vi "Panel.vi"(11 "ExBlank in":refnum<class "ExBlank.lvclass">) -> ()   [LabVIEW 2020, in "2D Array Example.lvlib" / "ExBlank.lvclass"]
uses:
  ExBlank.lvclass
  C:/dev/lv20CE/lv-oopanel/OOPanel/Panel/Panel.lvclass
  OOPanel/Panel/Basic UI State.ctl
  OOPanel/Panel/Panel.lvclass
  OOPanel/OOPanel.lvlib
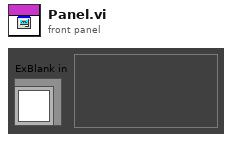
[diagram p1: front panel]
types:
  T1 = typedef "OOPanel.lvlib/Panel.lvclass/Basic UI State.ctl" = enum16{"Init", "Run", "Close"}
  T2 = typedef "OOPanel.lvlib/Panel.lvclass/Panel Events.ctl" = cluster{"Visbility":refnum<user-event>, "Close":refnum<user-event>}
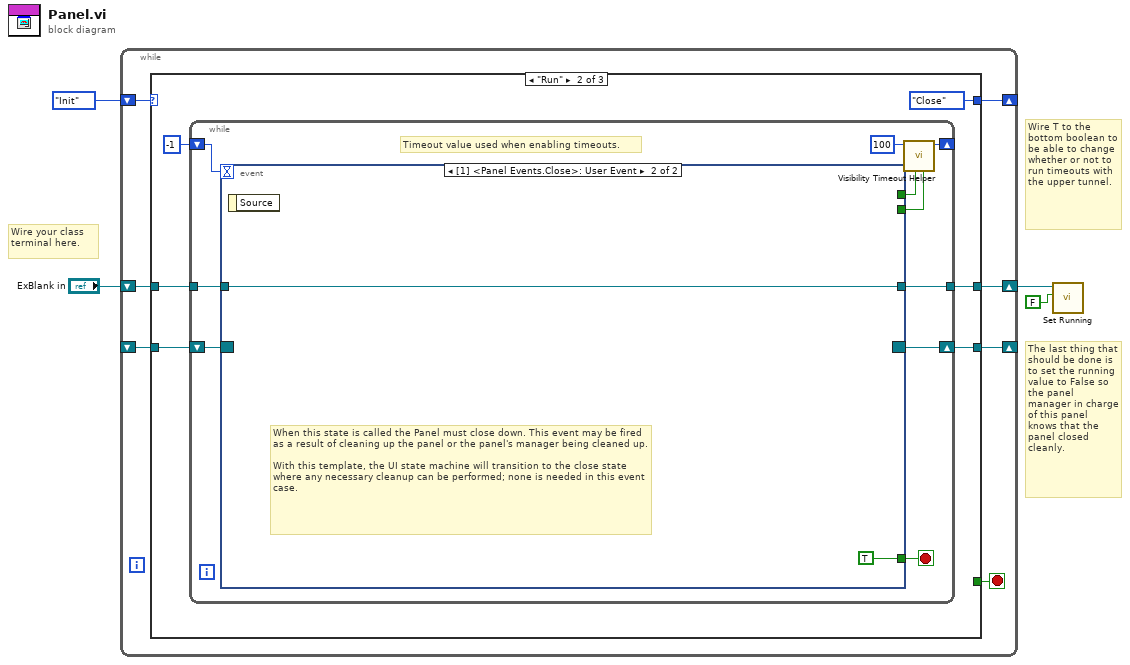
[diagram p0: block diagram]
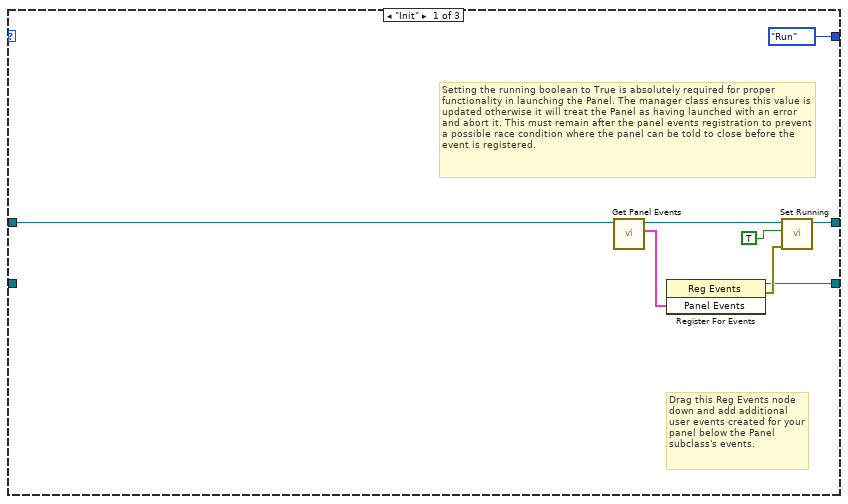
[diagram p2: hidden frame]
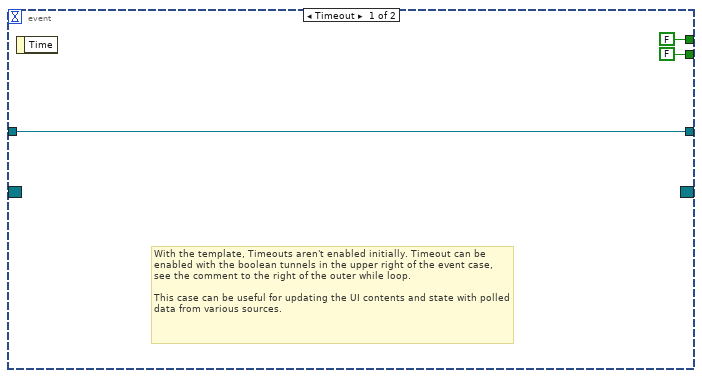
[diagram p3: hidden frame]
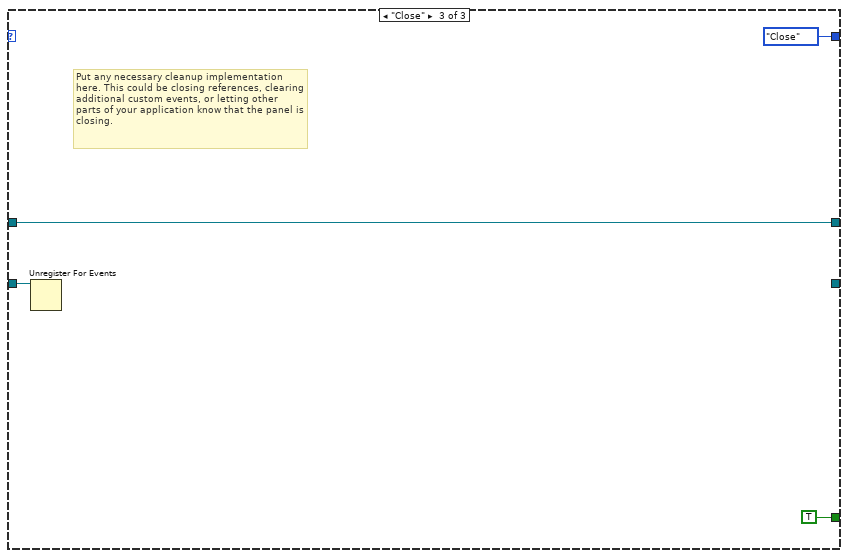
[diagram p4: hidden frame]
diagram:
  # "The last thing that should be done is to set the running value to False so the panel manager in charge of this panel knows that the panel closed cleanly."
  # "Wire T to the bottom boolean to be able to change whether or not to run timeouts with the upper tunnel."
  # "Wire your class terminal here."
  n1 = while {
    shift-right: [w10] -> _
    shift-left: _ -> [w11]
    shift-right: [w8] -> _
    shift-left: Basic_UI_State."Init" ("Basic UI State") -> [w9]
    shift-right: [w6] -> w4
    shift-left: "ExBlank in" -> [w5]
    stop <- w7 stop-if-true
    n2 = case shown="\"Run\"" w9 {
      tunnel: w11 -> [_ w25 w42]
      tunnel: [w16 w23 _] -> w10
      tunnel: [Basic_UI_State."Run" ("Basic UI State") Basic_UI_State."Close" ("Basic UI State") Basic_UI_State."Close" ("Basic UI State")] -> w8
      tunnel: [_ _ TRUE] -> w7
      tunnel: [w15 w20 w41] -> w6
      tunnel: w5 -> [w14 w21 w41]
      frame "Init" {
        # "Setting the running boolean to True is absolutely required for proper functionality in launching the Panel. The manager class ensures this value is updated otherwise it will treat the Panel as having launched with an error and abort it. This must remain after the panel events registration to prevent a possible race condition where the panel can be told to close before the event is registered."
        # "Drag this Reg Events node down and add additional user events created for your panel below the Panel subclass's events."
        n3 = call "Get Panel Events.vi"("Panel in"=w14) -> ("Panel Events"=w12:T2, "Panel out"=w13:refnum<class "ExBlank.lvclass">)  [unwired: 8 in, 1 out]
        n4 = register-events(w12) -> (reference out=w16:refnum<event-registration>, error out=w18:errorcluster)  [unwired: 2 in]
        n5 = call "Set Running.vi"("error in (no error)"=w18, "Running"=TRUE, "Panel in"=w13) -> ("Panel out"=w15:refnum<class "ExBlank.lvclass">)  [unwired: 7 in, 1 out]
      }
      frame "Run" {
        n6 = while {
          shift-right: [w31] -> w23
          shift-left: w25 -> [w32]
          shift-right: [w34] -> _
          shift-left: -1 ("Timeout") -> [w33]
          tunnel: w21 -> [w27]
          tunnel: [w26] -> w20
          stop <- w28 stop-if-true
          # "Timeout value used when enabling timeouts."
          n7 = event shown="[1] <Panel Events.Close>: User Event" {
            selector: w32 -> [_ _]
            dyn-events: [_ _] -> w31
            timeout: w33 -> [_ _]
            tunnel: [FALSE _] -> w30
            tunnel: [FALSE _] -> w29
            tunnel: [_ TRUE] -> w28
            tunnel: w27 -> [w36 w39]
            tunnel: [w36 w39] -> w26
            event Timeout {
              # "With the template, Timeouts aren't enabled initially. Timeout can be enabled with the boolean tunnels in the upper right of the event case, see the comment to the right of the outer while loop.\n\nThis case can be useful for updating the UI contents and state with polled data from various sources."
              n8 = event-data() -> ()  [unwired: 1 in, 1 out]
            }
            event User Event {
              # "When this state is called the Panel must close down. This event may be fired as a result of cleaning up the panel or the panel's manager being cleaned up.\n\nWith this template, the UI state machine will transition to the close state where any necessary cleanup can be performed; none is needed in this event case."
              n9 = event-data() -> ()  [unwired: 1 in, 1 out]
            }
          }
          n10 = call "Visibility Timeout Helper.vi"("Update?"=w29, "Use Timeout?"=w30, "Visible Timeout mS"=100) -> ("Timeout"=w34:i32)  [unwired: 8 in]
        }
      }
      frame "Close" {
        # "Put any necessary cleanup implementation here. This could be closing references, clearing additional custom events, or letting other parts of your application know that the panel is closing."
        n11 = Unregister For Events(event registration refnum=w42) -> ()  [unwired: 1 in, 1 out]
      }
    }
  }
  n12 = call "Set Running.vi"("Running"=FALSE, "Panel in"=w4) -> ()  [unwired: 8 in, 2 out]
